vi "Set Tuner Gain.vi"(8 "error in (no error)":errorcluster, 10 "Gain (dB)":dbl, 11 "RTL-SDR in":refnum<class "RTL-SDR.lvclass">) -> (0 "error out":errorcluster, 1 "function return":i32, 3 "RTL-SDR out":refnum<class "RTL-SDR.lvclass">)   [LabVIEW 2015, in "RTL-SDR.lvclass"]
uses:
  RTL-SDR.lvclass
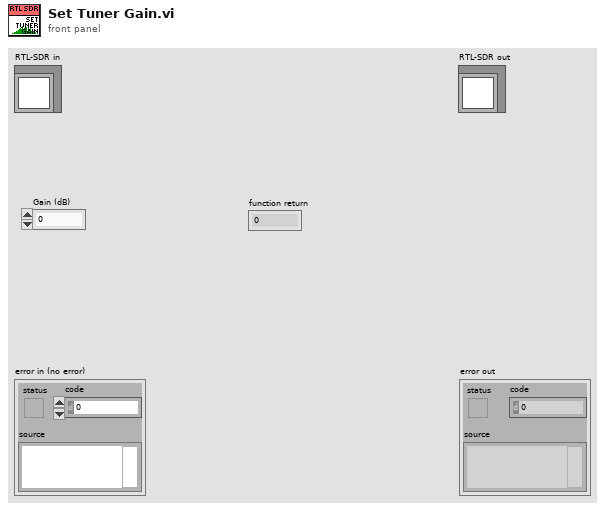
[diagram p1: front panel]
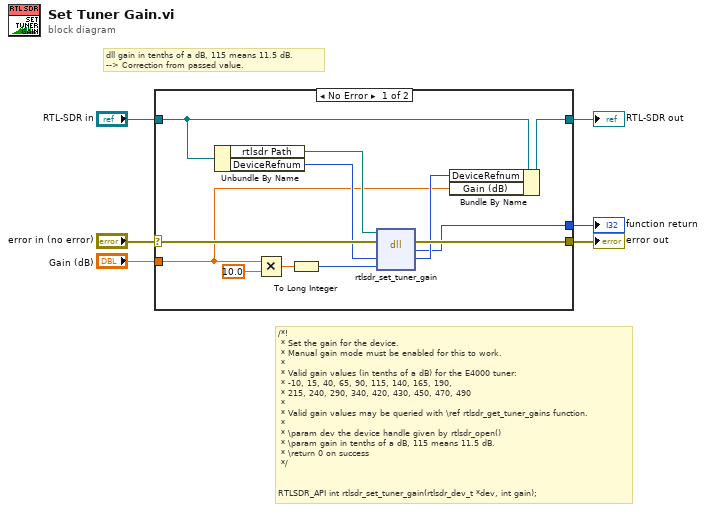
[diagram p0: block diagram]
diagram:
  # "dll gain in tenths of a dB, 115 means 11.5 dB. \n--> Correction from passed value."
  # "/*!\n * Set the gain for the device.\n * Manual gain mode must be enabled for this to work.\n *\n * Valid gain values (in tenths of a dB) for the E4000 tuner:\n * -10, 15, 40, 65, 90, 115, 140, 165, 190,\n * 215, 240, 290, 340, 420, 430, 450, 470, 490\n *\n * Valid gain values may be queried with \\ref rtlsdr_get_tuner_gains function.\n *\n * \\param dev the device handle given by rtlsdr_open()\n * \\param gain in tenths of a dB, 115 means 11.5 dB.\n * \\return 0 on success\n */\n\n\nRTLSDR_API int rtlsdr_set_tuner_gain(rtlsdr_dev_t *dev, int gain);"
  n1 = case shown="No Error" "error in (no error)" {
    selector: "error in (no error)" -> [w18 w20]
    tunnel: [w17 w20] -> w5
    tunnel: [w13 w19] -> w3
    tunnel: "RTL-SDR in" -> [w16 w19]
    tunnel: [w11 _] -> w2
    tunnel: "Gain (dB)" -> [w7 _]
    frame No Error {
      n2 = Unbundle By Name(w16) -> ("rtlsdr Path"=w15:path, "DeviceRefnum"=w14:u64)
      n3 = Multiply(x=w7, y=10.0) -> (x*y=w10:dbl)
      n4 = To Long Integer(number=w10) -> (32bit integer=w8:i32)
      n5 = dll-call lib="C:/Users/Ivan/Desktop/D-23-09-24 (RTL-SDR)/Project (Pelleng-SDR)/RTL-SDR Class/dll/rtlsdr.*" fn="rtlsdr_set_tuner_gain"(path in=w15, error in=w18, "DeviceRefnum"=w14, "Gain"=w8) -> (error out=w17:errorcluster, "return type"=w11:i32, "DeviceRefnum"=w12:u64)  [unwired: 2 in, 1 out]
      n6 = Bundle By Name(cluster=w16, "DeviceRefnum"=w12, "Gain (dB)"=w7) -> (w13:refnum<class "RTL-SDR.lvclass">)
    }
    frame Error {
    }
  }
  "error out" <- w5
  "RTL-SDR out" <- w3
  "function return" <- w2
